vi "Unpack Boolean.vi"(11 "Broadcast Boolean Msg In":refnum<class "Broadcast Boolean Msg.lvclass">) -> (2 "NewVal":bool, 3 "Control Label":string)   [LabVIEW 2015, in "Broadcast Boolean Msg.lvclass"]
uses:
  Broadcast Boolean Msg.lvclass
  Broadcast Boolean Msg.lvclass/Broadcast Boolean Msg.ctl
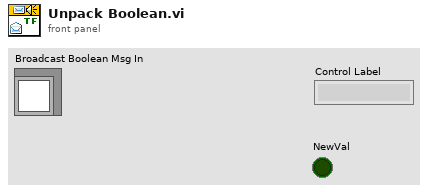
[diagram p1: front panel]
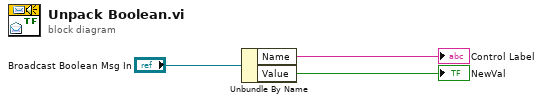
[diagram p0: block diagram]
diagram:
  n1 = Unbundle By Name("Broadcast Boolean Msg In") -> ("Name"=→"Control Label":string, "Value"=→"NewVal":bool)
